vi "Packet Strings to Values.vi"(11 "Pakcet Values":string[](array[string])) -> (3 "Data Report":T1)   [LabVIEW 2013]
uses:
  Payload Status.ctl
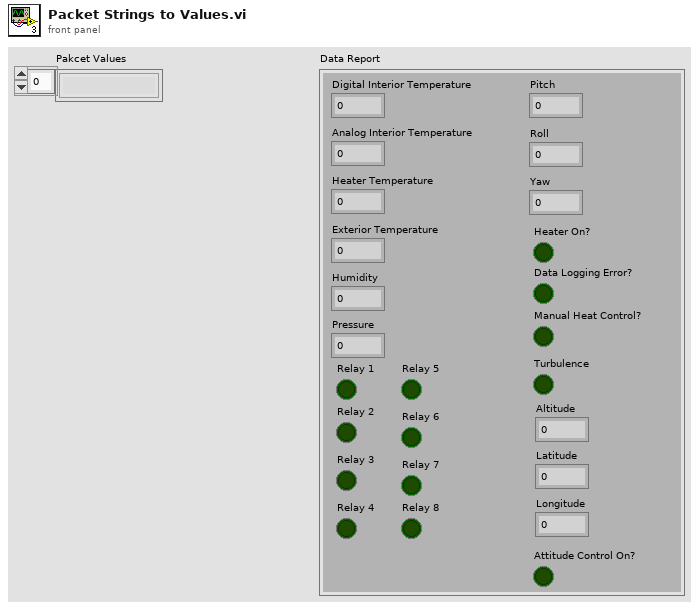
[diagram p1: front panel]
types:
  T1 = typedef "Payload Status.ctl" = cluster{"Digital Interior Temperature":dbl, "Analog Interior Temperature":dbl, "Heater Temperature":dbl, "Exterior Temperature":dbl, "Humidity":dbl, "Pressure":dbl, "Pitch":dbl, "Roll":dbl, "Yaw":dbl, "Heater On?":bool, "Data Logging Error?":bool, "Manual Heat Control?":bool, "Turbulence":bool, "Relay 1":bool, "Relay 2":bool, "Relay 3":bool, "Relay 4":bool, "Relay 5":bool, "Relay 6":bool, "Relay 7":bool, "Relay 8":bool, "Altitude":dbl, "Latitude":dbl, "Longitude":dbl, "Attitude Control On?":bool}
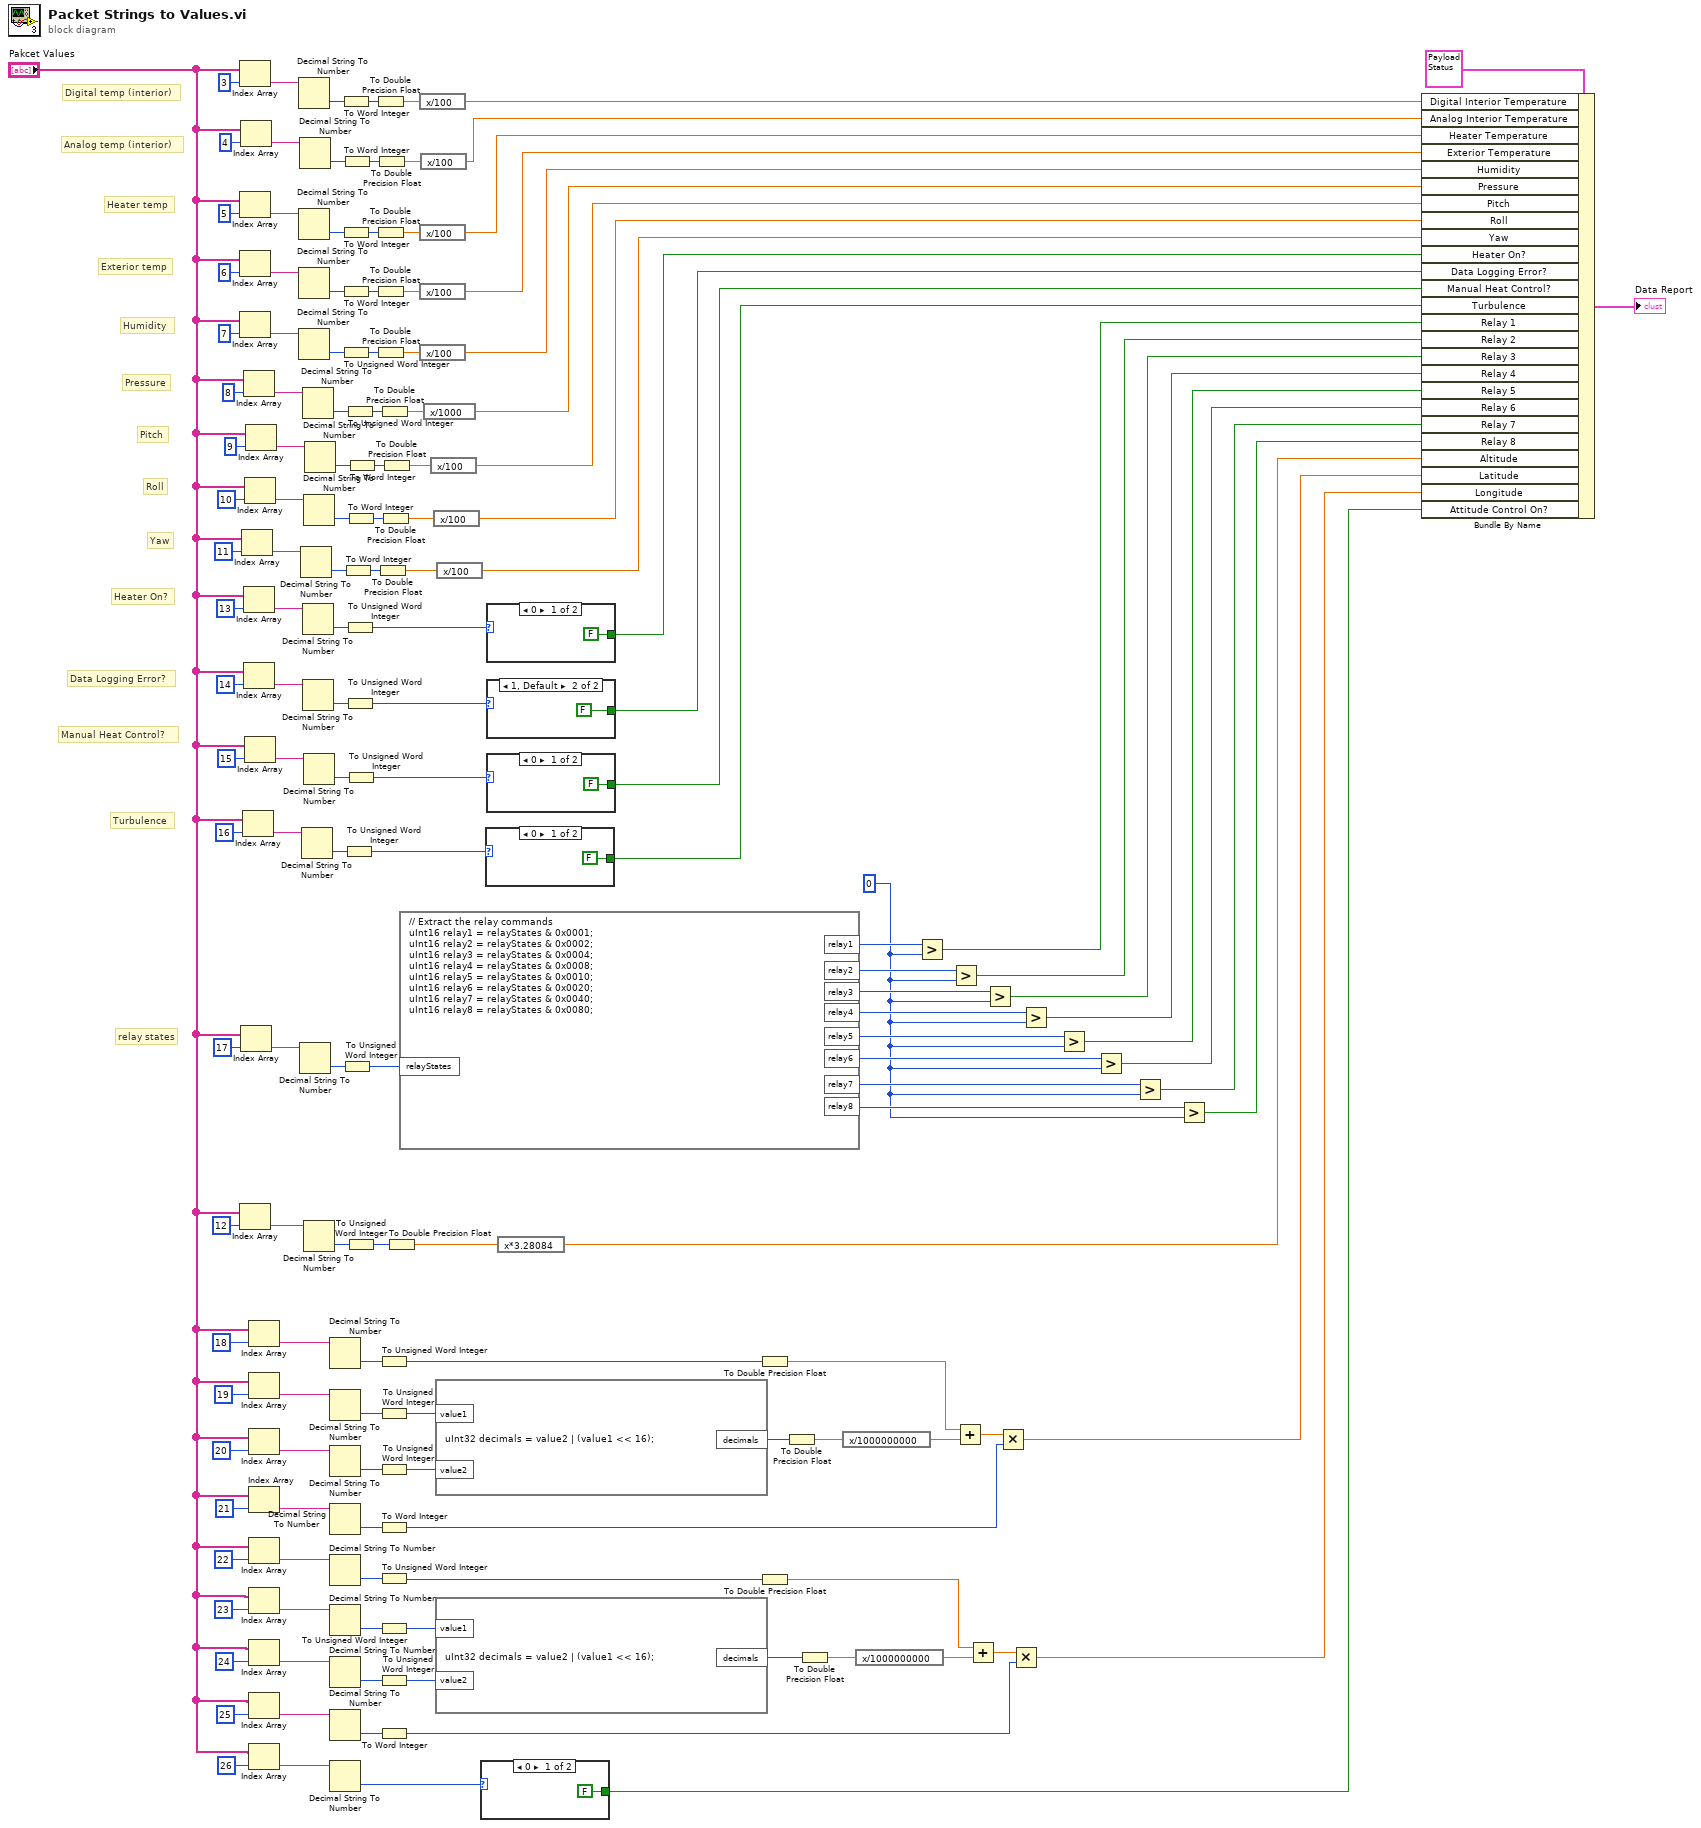
[diagram p0: block diagram]
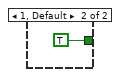
[diagram p2: hidden frame]
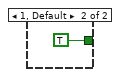
[diagram p3: hidden frame]
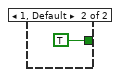
[diagram p4: hidden frame]
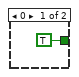
[diagram p5: hidden frame]
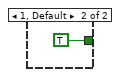
[diagram p6: hidden frame]
diagram:
  w3 = 0
  # "relay states"
  # "Turbulence"
  # "Manual Heat Control?"
  # "Data Logging Error?"
  # "Heater On?"
  # "Yaw"
  # "Roll"
  # "Pitch"
  # "Pressure"
  # "Humidity"
  # "Exterior temp"
  # "Heater temp"
  # "Analog temp (interior)"
  # "Digital temp (interior)"
  n1 = Index Array(array="Pakcet Values", index=3) -> (element=w150:string)
  n2 = Index Array(array="Pakcet Values", index=5) -> (element=w140:string)
  n3 = Index Array(array="Pakcet Values", index=6) -> (element=w135:string)
  n4 = Index Array(array="Pakcet Values", index=7) -> (element=w130:string)
  n5 = Index Array(array="Pakcet Values", index=12) -> (element=w63:string)
  n6 = Index Array(array="Pakcet Values", index=4) -> (element=w145:string)
  n7 = Index Array(array="Pakcet Values", index=17) -> (element=w82:string)
  n8 = Index Array(array="Pakcet Values", index=11) -> (element=w112:string)
  n9 = Index Array(array="Pakcet Values", index=16) -> (element=w87:string)
  n10 = Index Array(array="Pakcet Values", index=8) -> (element=w125:string)
  n11 = Index Array(array="Pakcet Values", index=13) -> (element=w108:string)
  n12 = Index Array(array="Pakcet Values", index=14) -> (element=w105:string)
  n13 = Index Array(array="Pakcet Values", index=10) -> (element=w116:string)
  n14 = Index Array(array="Pakcet Values", index=15) -> (element=w92:string)
  n15 = Index Array(array="Pakcet Values", index=9) -> (element=w120:string)
  n16 = Index Array(array="Pakcet Values", index=18) -> (element=w40:string)
  n17 = Index Array(array="Pakcet Values", index=19) -> (element=w39:string)
  n18 = Index Array(array="Pakcet Values", index=20) -> (element=w38:string)
  n19 = Index Array(array="Pakcet Values", index=21) -> (element=w42:string)
  n20 = Index Array(array="Pakcet Values", index=22) -> (element=w37:string)
  n21 = Index Array(array="Pakcet Values", index=23) -> (element=w36:string)
  n22 = Index Array(array="Pakcet Values", index=24) -> (element=w35:string)
  n23 = Index Array(array="Pakcet Values", index=25) -> (element=w34:string)
  n24 = Index Array(array="Pakcet Values", index=26) -> (element=w33:string)
  n25 = Decimal String To Number(string=w150) -> (number=w151:i32)  [unwired: 2 in, 1 out]
  n26 = Decimal String To Number(string=w140) -> (number=w141:i32)  [unwired: 2 in, 1 out]
  n27 = Decimal String To Number(string=w135) -> (number=w136:i32)  [unwired: 2 in, 1 out]
  n28 = Decimal String To Number(string=w130) -> (number=w131:i32)  [unwired: 2 in, 1 out]
  n29 = Decimal String To Number(string=w145) -> (number=w146:i32)  [unwired: 2 in, 1 out]
  n30 = Decimal String To Number(string=w82) -> (number=w83:i32)  [unwired: 2 in, 1 out]
  n31 = Decimal String To Number(string=w112) -> (number=w113:i32)  [unwired: 2 in, 1 out]
  n32 = Decimal String To Number(string=w87) -> (number=w88:i32)  [unwired: 2 in, 1 out]
  n33 = Decimal String To Number(string=w125) -> (number=w126:i32)  [unwired: 2 in, 1 out]
  n34 = Decimal String To Number(string=w108) -> (number=w109:i32)  [unwired: 2 in, 1 out]
  n35 = Decimal String To Number(string=w105) -> (number=w106:i32)  [unwired: 2 in, 1 out]
  n36 = Decimal String To Number(string=w116) -> (number=w117:i32)  [unwired: 2 in, 1 out]
  n37 = Decimal String To Number(string=w92) -> (number=w93:i32)  [unwired: 2 in, 1 out]
  n38 = Decimal String To Number(string=w63) -> (number=w64:i32)  [unwired: 2 in, 1 out]
  n39 = Decimal String To Number(string=w120) -> (number=w121:i32)  [unwired: 2 in, 1 out]
  n40 = Decimal String To Number(string=w40) -> (number=w32:i32)  [unwired: 2 in, 1 out]
  n41 = Decimal String To Number(string=w39) -> (number=w31:i32)  [unwired: 2 in, 1 out]
  n42 = Decimal String To Number(string=w38) -> (number=w30:i32)  [unwired: 2 in, 1 out]
  n43 = Decimal String To Number(string=w42) -> (number=w41:i32)  [unwired: 2 in, 1 out]
  n44 = Decimal String To Number(string=w37) -> (number=w29:i32)  [unwired: 2 in, 1 out]
  n45 = Decimal String To Number(string=w36) -> (number=w28:i32)  [unwired: 2 in, 1 out]
  n46 = Decimal String To Number(string=w35) -> (number=w27:i32)  [unwired: 2 in, 1 out]
  n47 = Decimal String To Number(string=w34) -> (number=w26:i32)  [unwired: 2 in, 1 out]
  n48 = Decimal String To Number(string=w33) -> (number=w25:i32)  [unwired: 2 in, 1 out]
  n49 = To Word Integer(number=w151) -> (16bit integer=w149:i16)
  n50 = To Word Integer(number=w141) -> (16bit integer=w139:i16)
  n51 = To Word Integer(number=w136) -> (16bit integer=w134:i16)
  n52 = To Unsigned Word Integer(number=w131) -> (unsigned 16bit integer=w129:u16)
  n53 = To Word Integer(number=w146) -> (16bit integer=w144:i16)
  n54 = To Unsigned Word Integer(number=w83) -> (unsigned 16bit integer=w81:u16)
  n55 = To Word Integer(number=w113) -> (16bit integer=w111:i16)
  n56 = To Unsigned Word Integer(number=w88) -> (unsigned 16bit integer=w86:u16)
  n57 = To Unsigned Word Integer(number=w126) -> (unsigned 16bit integer=w124:u16)
  n58 = To Unsigned Word Integer(number=w109) -> (unsigned 16bit integer=w98:u16)
  n59 = To Unsigned Word Integer(number=w106) -> (unsigned 16bit integer=w96:u16)
  n60 = To Word Integer(number=w117) -> (16bit integer=w115:i16)
  n61 = To Unsigned Word Integer(number=w93) -> (unsigned 16bit integer=w91:u16)
  n62 = To Unsigned Word Integer(number=w64) -> (unsigned 16bit integer=w54:u16)
  n63 = To Word Integer(number=w121) -> (16bit integer=w119:i16)
  n64 = To Double Precision Float(number=w149) -> (double precision float=w148:dbl)
  n65 = To Double Precision Float(number=w139) -> (double precision float=w138:dbl)
  n66 = To Double Precision Float(number=w134) -> (double precision float=w133:dbl)
  n67 = To Double Precision Float(number=w129) -> (double precision float=w128:dbl)
  n68 = To Double Precision Float(number=w144) -> (double precision float=w143:dbl)
  n69 = To Double Precision Float(number=w111) -> (double precision float=w59:dbl)
  n70 = To Unsigned Word Integer(number=w32) -> (unsigned 16bit integer=w22:u16)
  n71 = To Unsigned Word Integer(number=w31) -> (unsigned 16bit integer=w24:u16)
  n72 = To Unsigned Word Integer(number=w30) -> (unsigned 16bit integer=w23:u16)
  n73 = To Word Integer(number=w41) -> (16bit integer=w20:i16)
  n74 = To Unsigned Word Integer(number=w29) -> (unsigned 16bit integer=w18:u16)
  n75 = To Unsigned Word Integer(number=w28) -> (unsigned 16bit integer=w17:u16)
  n76 = To Unsigned Word Integer(number=w27) -> (unsigned 16bit integer=w16:u16)
  n77 = To Word Integer(number=w26) -> (16bit integer=w5:i16)
  n78 = To Double Precision Float(number=w124) -> (double precision float=w123:dbl)
  n79 = To Double Precision Float(number=w115) -> (double precision float=w60:dbl)
  n80 = To Double Precision Float(number=w119) -> (double precision float=w62:dbl)
  n81 = To Double Precision Float(number=w54) -> (double precision float=w2:dbl)
  n82 = formula code="// Extract the relay commands\nuInt16 relay1 = relayStates & 0x0001;\nuInt16 relay2 = relayStates & 0x0002;\nuInt16 relay3 = relayStates & 0x0004;\nuInt16 relay4 = relayStates & 0x0008;\nuInt16 relay5 = relayStates & 0x0010;\nuInt16 relay6 = relayStates & 0x0020;\nuInt16 relay7 = relayStates & 0x0040;\nuInt16 relay8 = relayStates & 0x0080;"("relayStates"=w81) -> ("relay1"=w80:u16, "relay2"=w79:u16, "relay3"=w78:u16, "relay4"=w77:u16, "relay5"=w76:u16, "relay6"=w75:u16, "relay7"=w74:u16, "relay8"=w73:u16)
  n83 = expression code="x/100"(w148) -> (w104:dbl)
  n84 = expression code="x/100"(w138) -> (w102:dbl)
  n85 = expression code="x/100"(w133) -> (w101:dbl)
  n86 = expression code="x/100"(w128) -> (w100:dbl)
  n87 = expression code="x/100"(w143) -> (w103:dbl)
  n88 = expression code="x/1000"(w123) -> (w99:dbl)
  n89 = expression code="x/100"(w62) -> (w61:dbl)
  n90 = expression code="x/100"(w60) -> (w57:dbl)
  n91 = formula code="uInt32 decimals = value2 | (value1 << 16);"("value1"=w24, "value2"=w23) -> ("decimals"=w13:u32)
  n92 = formula code="uInt32 decimals = value2 | (value1 << 16);"("value1"=w17, "value2"=w16) -> ("decimals"=w6:u32)
  n93 = expression code="x/100"(w59) -> (w58:dbl)
  n94 = case shown="0" w25 {
    tunnel: [FALSE TRUE] -> w14
    frame 0 {
    }
    frame 1, Default {
    }
  }
  n95 = case shown="0" w86 {
    tunnel: [FALSE TRUE] -> w85
    frame 0 {
    }
    frame 1, Default {
    }
  }
  n96 = case shown="0" w98 {
    tunnel: [FALSE TRUE] -> w97
    frame 0 {
    }
    frame 1, Default {
    }
  }
  n97 = case shown="1, Default" w96 {
    tunnel: [TRUE FALSE] -> w95
    frame 0 {
    }
    frame 1, Default {
    }
  }
  n98 = case shown="0" w91 {
    tunnel: [FALSE TRUE] -> w90
    frame 0 {
    }
    frame 1, Default {
    }
  }
  n99 = expression code="x*3.28084"(w2) -> (w1:dbl)
  n100 = To Double Precision Float(number=w22) -> (double precision float=w19:dbl)
  n101 = To Double Precision Float(number=w18) -> (double precision float=w7:dbl)
  n102 = To Double Precision Float(number=w13) -> (double precision float=w12:dbl)
  n103 = To Double Precision Float(number=w6) -> (double precision float=w9:dbl)
  n104 = expression code="x/1000000000"(w12) -> (w11:dbl)
  n105 = expression code="x/1000000000"(w9) -> (w8:dbl)
  n106 = Greater?(x=w80, y=w3) -> (0:w66:bool)
  n107 = Greater?(x=w79, y=w3) -> (0:w53:bool)
  n108 = Add(x=w19, y=w11) -> (x+y=w21:dbl)
  n109 = Add(x=w7, y=w8) -> (x+y=w10:dbl)
  n110 = Greater?(x=w78, y=w3) -> (0:w67:bool)
  n111 = Multiply(x=w21, y=w20) -> (x*y=w15:dbl)
  n112 = Multiply(x=w10, y=w5) -> (x*y=w4:dbl)
  n113 = Greater?(x=w77, y=w3) -> (0:w68:bool)
  n114 = Greater?(x=w76, y=w3) -> (0:w69:bool)
  n115 = Greater?(x=w75, y=w3) -> (0:w70:bool)
  n116 = Greater?(x=w74, y=w3) -> (0:w71:bool)
  n117 = Greater?(x=w73, y=w3) -> (0:w72:bool)
  n118 = Bundle By Name(cluster=T1 {"Digital Interior Temperature"=0.0, "Analog Interior Temperature"=0.0, "Heater Temperature"=0.0, "Exterior Temperature"=0.0, "Humidity"=0.0, "Pressure"=0.0, "Pitch"=0.0, "Roll"=0.0, "Yaw"=0.0, "Heater On?"=FALSE, "Data Logging Error?"=FALSE, "Manual Heat Control?"=FALSE, "Turbulence"=FALSE, "Relay 1"=FALSE, "Relay 2"=FALSE, "Relay 3"=FALSE, "Relay 4"=FALSE, "Relay 5"=FALSE, "Relay 6"=FALSE, "Relay 7"=FALSE, "Relay 8"=FALSE, "Altitude"=0.0, "Latitude"=0.0, "Longitude"=0.0, "Attitude Control On?"=FALSE} ("Data Report"), "Digital Interior Temperature"=w104, "Analog Interior Temperature"=w103, "Heater Temperature"=w102, "Exterior Temperature"=w101, "Humidity"=w100, "Pressure"=w99, "Pitch"=w61, "Roll"=w57, "Yaw"=w58, "Heater On?"=w97, "Data Logging Error?"=w95, "Manual Heat Control?"=w90, "Turbulence"=w85, "Relay 1"=w66, "Relay 2"=w53, "Relay 3"=w67, "Relay 4"=w68, "Relay 5"=w69, "Relay 6"=w70, "Relay 7"=w71, "Relay 8"=w72, "Altitude"=w1, "Latitude"=w15, "Longitude"=w4, "Attitude Control On?"=w14) -> (→"Data Report":T1)
